vi "loginLimit.vi"(8 "error in (no error)":errorcluster caption="错误输入（无错误）") -> (0 "error out":errorcluster caption="错误输出", 3 "true":bool)   [LabVIEW 2014]
panel:
  in  "取消":bool
  in  "确定":bool
  in  "密码":string
  out "用户名":string="admin"
  # "请输入密码"
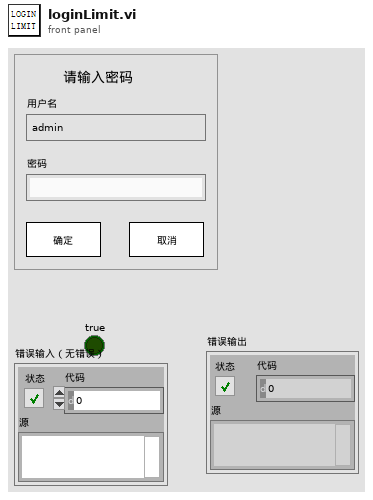
[diagram p1: front panel]
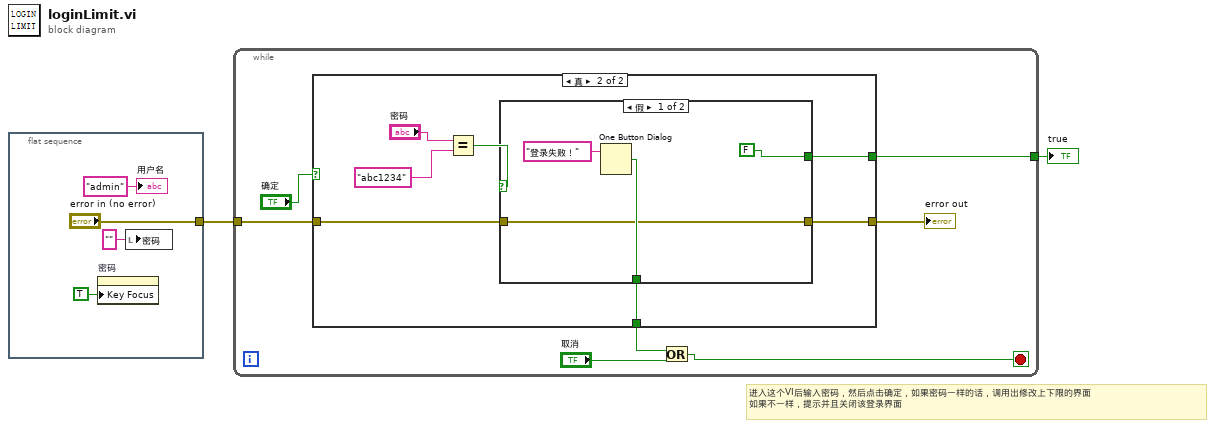
[diagram p0: block diagram]
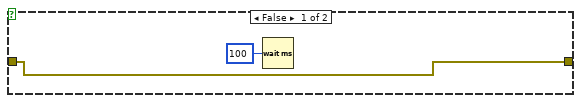
[diagram p2: hidden frame]
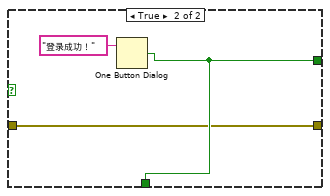
[diagram p3: hidden frame]
diagram:
  # "进入这个VI后输入密码，然后点击确定，如果密码一样的话，调用出修改上下限的界面\n如果不一样，提示并且关闭该登录界面"
  n1 = flat-sequence {
    tunnel: ["error in (no error)"] -> w1
    frame #0 {
      n2 = property on="密码" class="Str"("Key Focus"=TRUE ("键选中")) -> ()  [unwired: 2 in, 2 out]
      n3 = local write "密码"("" ("密码")) -> ()
      "用户名" <- "admin" ("用户名")
    }
  }
  n4 = while {
    tunnel: [w12] -> w2
    tunnel: w1 -> [w8]
    stop <- w9 stop-if-true
    n5 = case shown="真" "确定" {
      tunnel: [_ w19] -> w12
      tunnel: [_ w18] -> w11
      tunnel: w8 -> [w14 w17]
      tunnel: [w14 w16] -> w7
      frame False {
        n6 = Wait (ms)(milliseconds to wait=u32 100 ("等待时间（毫秒）")) -> ()  [unwired: 1 out]
      }
      frame True {
        n7 = Equal?(x="密码", y="abc1234") -> (x = y?=w20:bool)
        n8 = case shown="假" w20 {
          tunnel: [FALSE w28] -> w19
          tunnel: [w24 w28] -> w18
          tunnel: w17 -> [w23 w27]
          tunnel: [w23 w27] -> w16
          frame False {
            n9 = One Button Dialog(message="登录失败！" ("消息")) -> (true=w24:bool)  [unwired: 1 in]
          }
          frame True {
            n10 = One Button Dialog(message="登录成功！" ("消息")) -> (true=w28:bool)  [unwired: 1 in]
          }
        }
      }
    }
    "error out" <- w7
    n11 = Or(x=w11, y="取消") -> (x .or. y?=w9:bool)
  }
  "true" <- w2
